vi "Autotune PID.vi"(7 "Unit Address (1)":i16=1, 8 "error in (no error)":errorcluster {"code" format="%.0x"}, 9 "Channel 2 Autotune (0: Tune Off)":u16(ring) items=["Tune Off", "Ch2 PID Set 6", "Ch2 PID Set 7", "Ch2 PID Set 8", "Ch2 PID Set 9", "Ch2 PID Set 10"], 10 "Channel 1 Autotune (0: Tune Off)":u16(ring) items=["Tune Off", "Ch1 PID Set 1", "Ch1 PID Set 2", "Ch1 PID Set 3", "Ch1 PID Set 4", "Ch1 PID Set 5"], 11 "VISA resource name":refnum<visa-resource-name>) -> (0 "error out":errorcluster {"code" format="%.0x"}, 3 "VISA resource name out":refnum<visa-resource-name>)   [LabVIEW 2010]
doc: "This VI configures PID autotuning."
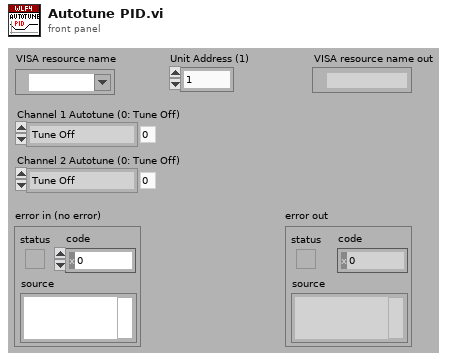
[diagram p1: front panel]
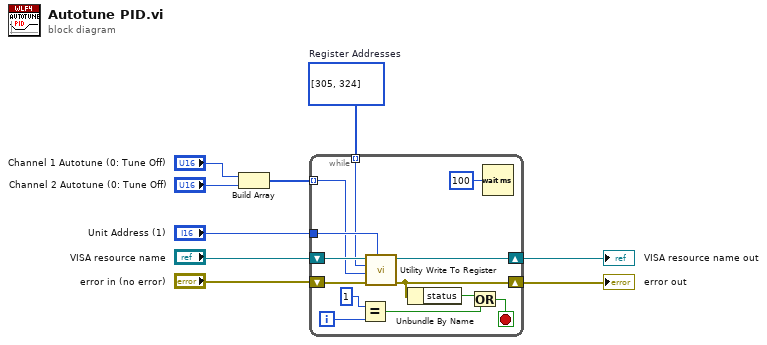
[diagram p0: block diagram]
diagram:
  w2 = i32[] [305, 324]  # Register Addresses
  n1 = Build Array("Channel 1 Autotune (0: Tune Off)", "Channel 2 Autotune (0: Tune Off)") -> (w1:u16[])
  n2 = while {
    shift-right: [w20] -> w5
    shift-left: "VISA resource name" -> [w22]
    shift-right: [w18] -> w6
    shift-left: "error in (no error)" -> [w21]
    tunnel: "Unit Address (1)" -> [w12]
    tunnel: w2 -> [w11] mode=indexing
    tunnel: w1 -> [w10] mode=indexing
    i -> [w14]
    stop <- w16 stop-if-true
    n3 = Equal?(x=1, y=w14) -> (x = y?=w13:bool)
    n4 = call "Utility Write To Register.vi"("Unit Address (1)"=w12, "error in (no error)"=w21, "Data (0)"=w10, "Register Address (0)"=w11, "VISA resource name"=w22) -> ("error out"=w18:errorcluster, "VISA resource name out"=w20:refnum<visa-resource-name>)  [unwired: 5 in]
    n5 = Unbundle By Name(w18) -> ("status"=w17:bool)
    n6 = Or(x=w17, y=w13) -> (x .or. y?=w16:bool)
    n7 = Wait (ms)(milliseconds to wait=u32 100) -> ()  [unwired: 1 out]
  }
  "error out" <- w6
  "VISA resource name out" <- w5
